vi "ProdaNG.Time.Get.vi"(7 "error in":errorcluster, 10 "dbHandleIn":i32) -> (0 "error out":errorcluster, 1 "time":timestamp, 2 "timeStr":string, 3 "dbHandle":i32)   [LabVIEW 2016]
doc: "This function passes back the current system time of the database.\nParameter:\nhandle is an Integer, that is returned by the function Login() when a new connection is created.\ntimeBuf is a Character Array in which the time given back in the format DD.MM.YYYY HH24:MI:SS when the Returncode is 0.\nReturncodes:\n0 No error\n< 0 ORACLE error code\n6 (ERROR_INVALID_HANDLE) in case of an invalid handle"
uses:
  prodllNG.dll
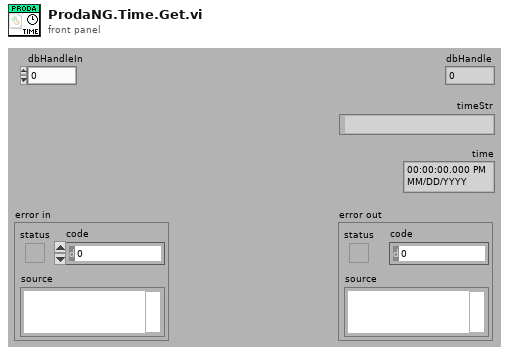
[diagram p1: front panel]
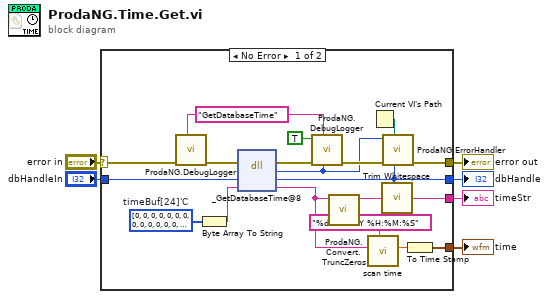
[diagram p0: block diagram]
diagram:
  n1 = case shown="No Error" "error in" {
    selector: "error in" -> [w18 w27]
    tunnel: [w24 w27] -> w5
    tunnel: "dbHandleIn" -> [w17 w26]
    tunnel: [w16 w26] -> w3
    tunnel: [w12 _] -> w2
    tunnel: [w7 _] -> w1
    frame No Error {
      w22 = "GetDatabaseTime" ("cmd")
      w25 = u8[] [0, 0, 0, 0, 0, 0, 0, 0, 0, 0, 0, 0, 0, 0, 0, 0, 0, 0, 0, 0, 0, 0, 0, 0]  # timeBuf[24]'C
      n2 = call "ProdaNG.DebugLogger.vi"("cmd"=w22, "error in (no error)"=w18) -> ("error out"=w21:errorcluster)  [unwired: 9 in]
      n3 = Byte Array To String(unsigned byte array=w25) -> (string=w11:string)
      n4 = dll-call lib="D:/svn/LineTraceSystem/SOFTWARE/sources/Database/ProdaNG/prodllNG.dll" fn="_GetDatabaseTime@8" ("ProDll.dll:Login")(error in=w21, "dbHandle"=w17, "timeBuf"=w11) -> (error out=w20:errorcluster, w15:i32, "dbHandle"=w16:i32, "timeBuf"=w10:string)  [unwired: 2 in, 1 out]
      n5 = call "ProdaNG.DebugLogger.vi"("return type"=w15, "cmd"=w22, "error in (no error)"=w20, "done? (F)"=TRUE) -> ("error out"=w19:errorcluster)  [unwired: 7 in]
      n6 = call "ProdaNG.Convert.TruncZeros.vi"("string with \\0s"=w10) -> ("LV string"=w13:string)  [unwired: 10 in]
      n7 = call "scan time.vi"("time format string"="%d.%m.%Y %H:%M:%S", "formatted time string"=w10) -> ("lv time (UTC)"=w8:dbl)  [unwired: 5 in, 4 out]
      n8 = Current VI's Path() -> (path=w23:path)
      n9 = call <vilib>:"Trim Whitespace.vi"("string"=w13) -> ("trimmed string"=w12:string)  [unwired: 1 in]
      n10 = call "ProdaNG.ErrorHandler.vi"("dbHandleIn"=w16, "Path"=w23, "error in"=w19, "output_parameter"=w15) -> ("error out"=w24:errorcluster)  [unwired: 7 in]
      n11 = To Time Stamp(1:w8) -> (0:w7:timestamp)
    }
    frame Error {
    }
  }
  "error out" <- w5
  "dbHandle" <- w3
  "timeStr" <- w2
  "time" <- w1
